vi "Set Record Length.vi"(7 "instance":i32, 8 "error in":errorcluster, 10 "record length":u32, 11 "lia host in":refnum<class "LIA Host Interface FPGA.lvclass">) -> (0 "error out":errorcluster, 3 "lia host out":refnum<class "LIA Host Interface FPGA.lvclass">)   [LabVIEW 2017, in "LIA Host Interface FPGA.lvclass"]
uses:
  LIA Host Interface FPGA.lvclass
  LIA Host Interface FPGA.lvclass/LIA Host Interface FPGA.ctl
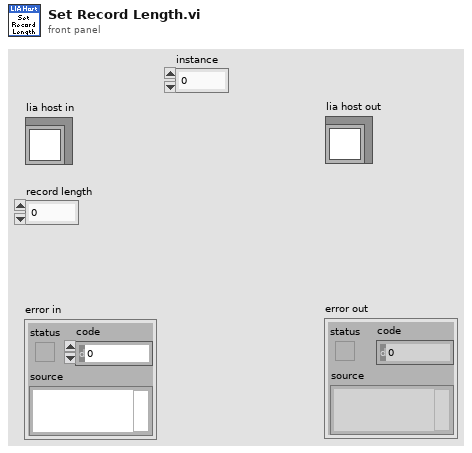
[diagram p1: front panel]
types:
  T1 = typedef "LIA Host Interface Desktop.lvclass/session data.ctl" = cluster{"fpga session":refnum<k20>, "record length":u32[]}
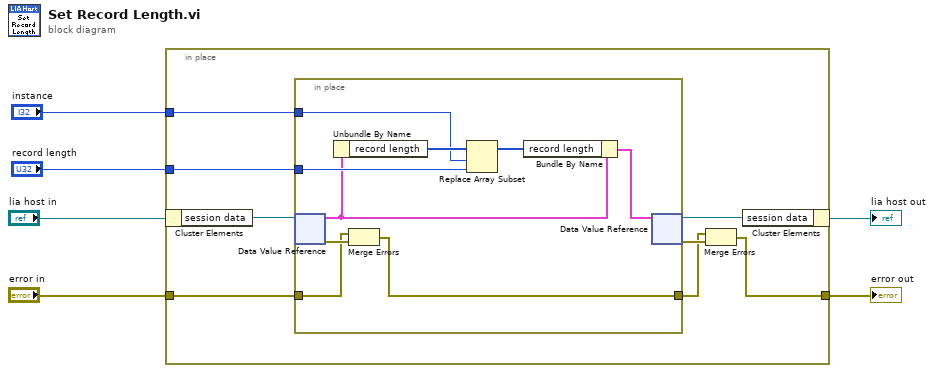
[diagram p0: block diagram]
diagram:
  n1 = in-place {
    in-place-border: "error in" -> [w12]
    in-place-border: [w9] -> w3
    in-place-border: "record length" -> [w8]
    in-place-border: "instance" -> [w7]
    n2 = in-place-cluster #1("lia host in") -> ("session data"=w14:refnum<data-value>)
    n3 = in-place {
      in-place-border: w12 -> [w22]
      in-place-border: [w21] -> w10
      in-place-border: w8 -> [w19]
      in-place-border: w7 -> [w18]
      n4 = in-place-dvr #2(w14) -> (w16:T1, w23:errorcluster)
      n5 = Unbundle By Name(w16) -> ("record length"=w20:u32[])
      n6 = Merge Errors(w22, w23) -> (w21:errorcluster)
      n7 = Replace Array Subset(array=w20, new element=w19, index=w18) -> (w17:u32[])
      n8 = Bundle By Name(cluster=w16, "record length"=w17) -> (w15:T1)
      n9 = in-place-dvr #2(w15) -> (w13:refnum<data-value>, w11:errorcluster)
    }
    n10 = Merge Errors(w10, w11) -> (w9:errorcluster)
    n11 = in-place-cluster #1("session data"=w13) -> (→"lia host out":refnum<class "LIA Host Interface FPGA.lvclass">)
  }
  "error out" <- w3
